vi "add tag to dictionary.vi"(8 "error in":errorcluster, 10 "system tag":refnum<class "data bus tag description.lvclass">, 11 "data dictionary in":refnum<class "data bus dictionary.lvclass">) -> (0 "error out":errorcluster, 3 "data dictionary out":refnum<class "data bus dictionary.lvclass">)   [LabVIEW 2013, in "data bus dictionary.lvclass"]
doc: "Adds a single tab to the data dictionary, including adding that tag to the default data table."
uses:
  data bus dictionary.lvclass
  tag/data bus tag description.lvclass
  tag/data bus tag description.lvclass/data bus tag description.ctl
  dictionary lookup value.ctl
  tag/Data Type.ctl
  data bus dictionary.lvclass/data bus dictionary.ctl
  table/add tag to table.vi
  tag/read default value.vi
  tag/read raw default value.vi
  tag/default value polymorphs/read default value Double.vi
  tag/default value polymorphs/read default value I64.vi
  tag/default value polymorphs/read default value Boolean.vi
  tag/default value polymorphs/read default value Array of Double.vi
  tag/default value polymorphs/read default value Array of I64.vi
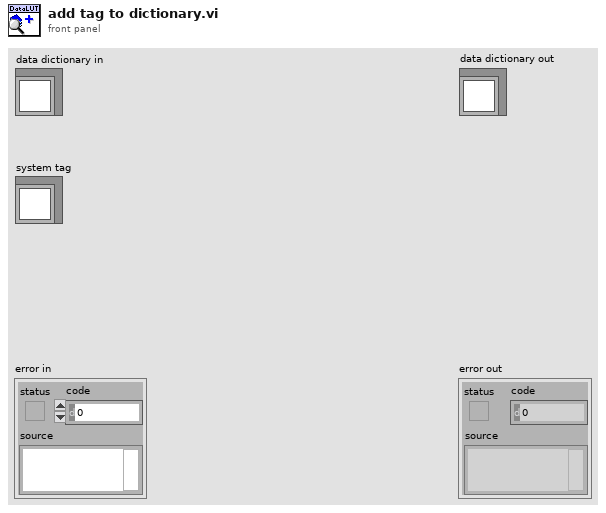
[diagram p1: front panel]
types:
  T1 = typedef "data bus dictionary.lvclass/dictionary lookup value.ctl" = cluster{"data type":T2, "index":i32}
  T2 = typedef "data bus tag description.lvclass/Data Type.ctl" = enum16{"Double", "I64", "Boolean", "Array of Double", "Array of I64", "Variant"}
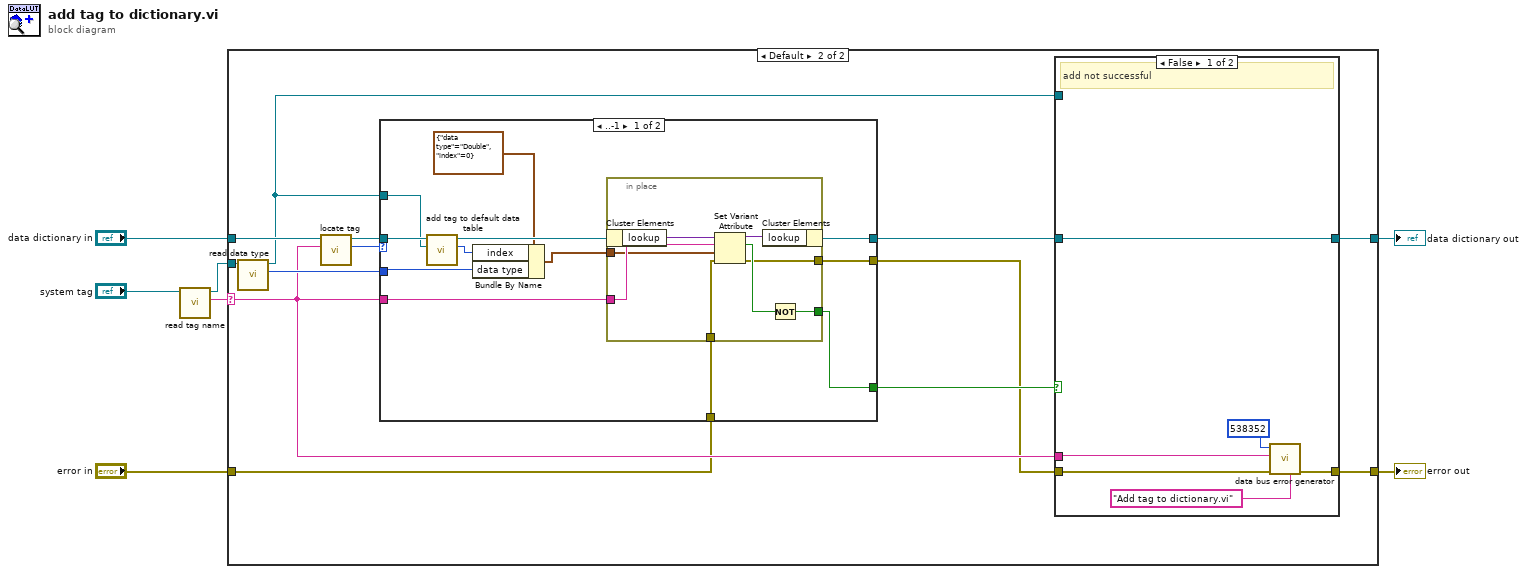
[diagram p0: block diagram]
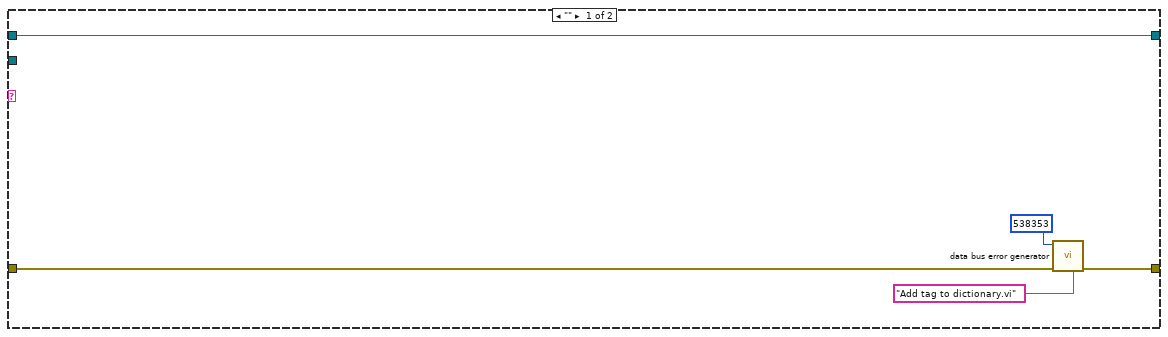
[diagram p2: hidden frame]
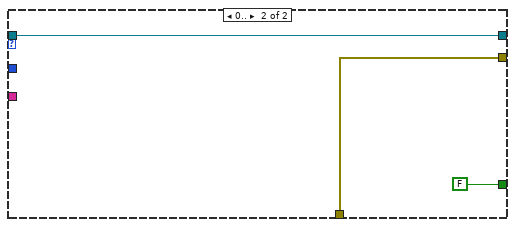
[diagram p4: hidden frame]
diagram:
  n1 = call "read tag name.vi"("system tag in"="system tag") -> ("name"=w1:string, "system tag out"=w3:refnum<class "data bus tag description.lvclass">)  [unwired: 8 in, 1 out]
  n2 = case shown="Default" w1 {
    selector: w1 -> [_ w16]
    tunnel: [w9 w25] -> w7
    tunnel: [w12 w23] -> w5
    tunnel: "error in" -> [w8 w14]
    tunnel: w3 -> [_ w21]
    tunnel: "data dictionary in" -> [w12 w20]
    frame "" {
      n3 = call "data bus error generator.vi"("error in"=w8, "source"="Add tag to dictionary.vi", "error code (0)"=538353) -> ("error out"=w9:errorcluster)  [unwired: 6 in]
    }
    frame Default {
      n4 = call "read data type.vi"("system tag in"=w21) -> ("data type"=w17:T2, "system tag out"=w15:refnum<class "data bus tag description.lvclass">)  [unwired: 8 in, 1 out]
      n5 = call "locate tag.vi"("name"=w16, "data dictionary in"=w20) -> ("index"=w18:i32, "data dictionary out"=w19:refnum<class "data bus dictionary.lvclass">)  [unwired: 6 in, 2 out]
      n6 = case shown="..-1" w18 {
        tunnel: w17 -> [w36 _]
        tunnel: w16 -> [w45 _]
        tunnel: w19 -> [w43 w56]
        tunnel: [w44 w56] -> w24
        tunnel: [w40 FALSE] -> w22
        tunnel: w15 -> [w41 _]
        tunnel: w14 -> [w39 w54]
        tunnel: [w38 w54] -> w13
        frame ..-1 {
          n7 = call "add tag to default data table.vi"("system tag"=w41, "data dictionary in"=w43) -> ("new index"=w35:i32, "data dictionary out"=w42:refnum<class "data bus dictionary.lvclass">)  [unwired: 7 in, 1 out]
          n8 = Bundle By Name(cluster=T1 {"data type"=enum."Double", "index"=0} ("dictionary lookup"), "index"=w35, "data type"=w36) -> (w34:T1)
          n9 = in-place {
            in-place-border: w45 -> [w47]
            in-place-border: [w50] -> w40
            in-place-border: w39 -> [w49]
            in-place-border: [w48] -> w38
            in-place-border: w34 -> [w46]
            n10 = in-place-cluster #1(w42) -> ("lookup"=w52:variant)
            n11 = Set Variant Attribute(Variant=w52, name=w47, value=w46, error in=w49) -> (Variant out=w53:variant, replaced=w51:bool, error out=w48:errorcluster)
            n12 = in-place-cluster #1("lookup"=w53) -> (w44:refnum<class "data bus dictionary.lvclass">)
            n13 = Not(x=w51) -> (.not. x?=w50:bool)
          }
        }
        frame 0.. {
        }
      }
      n14 = case shown="False" w22 {
        tunnel: w13 -> [w31 w32]
        tunnel: [w30 w32] -> w25
        tunnel: w16 -> [w28 _]
        tunnel: w24 -> [w27 w33]
        tunnel: [w27 w33] -> w23
        tunnel: w15 -> [_ _]
        frame False {
          # "add not successful"
          n15 = call "data bus error generator.vi"("error in"=w31, "source"="Add tag to dictionary.vi", "append error message"=w28, "error code (0)"=538352) -> ("error out"=w30:errorcluster)  [unwired: 5 in]
        }
        frame True {
          # "add succeeded"
        }
      }
    }
  }
  "error out" <- w7
  "data dictionary out" <- w5
